vi "RMXCommCheck.vi"(7 "Instrument Firmware Revision in":string, 8 "error in (no error)":errorcluster, 9 "Error Message":string, 10 "Instrument Driver Revision in":string, 11 "RMXInformation in":string) -> (0 "Error":bool, 1 "resulting string":string, 2 "Instrument Driver Revision out":string, 3 "Instrument Firmware Revision out":string, 4 "f":i32, 5 "RMXInformation out":string)   [LabVIEW 2023]
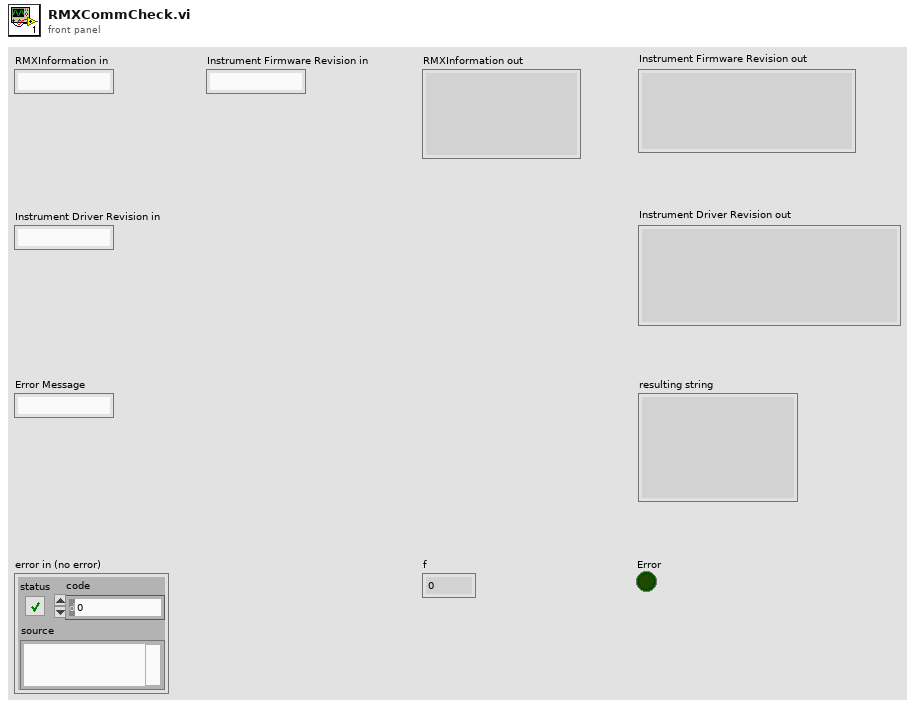
[diagram p1: front panel]
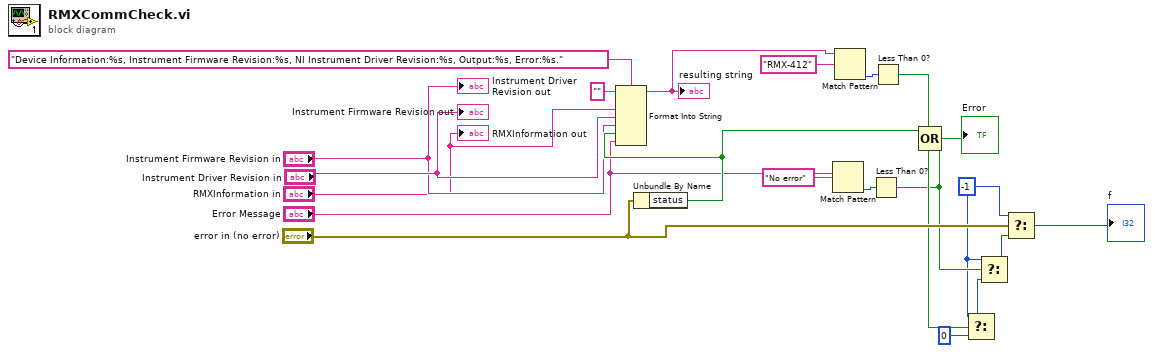
[diagram p0: block diagram]
diagram:
  w1 = -1 ("Status")
  n1 = Unbundle By Name("error in (no error)") -> ("status"=w21:bool)
  n2 = Format Into String(format string="Device Information:%s, Instrument Firmware Revision:%s, NI Instrument Driver Revision:%s, Output:%s, Error:%s.", initial string="", "RMXInformation in", "Instrument Driver Revision in", "Instrument Firmware Revision in", w21, "Error Message") -> (resulting string=w13:string)  [unwired: 1 in, 1 out]
  "resulting string" <- w13
  n3 = Match Pattern(string="Error Message", regular expression="No error" ("search string")) -> (offset past match=w10:i32)  [unwired: 1 in, 3 out]
  n4 = Match Pattern(string=w13, regular expression="RMX-412" ("search string")) -> (offset past match=w12:i32)  [unwired: 1 in, 3 out]
  n5 = Less Than 0?(x=w10) -> (x < 0?=w14:bool)
  n6 = Less Than 0?(x=w12) -> (x < 0?=w16:bool)
  n7 = Compound Arithmetic op=OR(w21, w14, w16) -> (→"Error":bool)
  n8 = Select(t=w1, s=w16, f=0) -> (s? t:f=w17:i32)
  n9 = Select(t=w1, s=w14, f=w17) -> (s? t:f=w15:i32)
  n10 = Select(t=w1, s="error in (no error)", f=w15) -> (s? t:f=→"f":i32)
  "Instrument Driver Revision out" <- "Instrument Firmware Revision in"
  "Instrument Firmware Revision out" <- "Instrument Driver Revision in"
  "RMXInformation out" <- "RMXInformation in"
